vi "Stop Core.vi"(10 "final error code":i32, 11 "Example Controller Actor In":refnum<class "Example Controller Actor.lvclass">) -> (3 "Example Controller Actor Out":refnum<class "Example Controller Actor.lvclass">)   [LabVIEW 2017, in "Example GUI View Actor.lvlib" / "Example Controller Actor.lvclass"]
doc: "(<B>Filename</B>: Actor Framework.lvlib:Actor.lvclass:Stop Core.vi)\n\nDefines what the actor does before it stops. Use the <B>final error code</B> input to determine whether the actor shut down in response to an error.\n\nBy default, this method does nothing. A descendant class may override it to define behavior, such as shutting down any processes the actor initiated in its override of the Actor Core method."
uses:
  Example Controller Actor.lvclass
  Example Controller Actor.lvclass/Example Controller Actor.ctl
  Example Controller Actor/Example Controller Actor/Example Controller Actor.lvclass
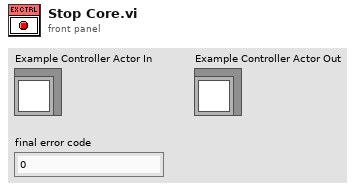
[diagram p1: front panel]
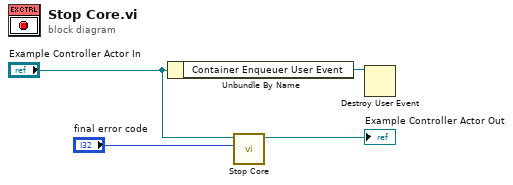
[diagram p0: block diagram]
diagram:
  n1 = Unbundle By Name("Example Controller Actor In") -> ("Container Enqueuer User Event"=w1:refnum<user-event>)
  n2 = call-parent "Stop Core.vi"("final error code"="final error code", "Controller Actor In"="Example Controller Actor In") -> ("Controller Actor Out"=→"Example Controller Actor Out":refnum<class "Example Controller Actor.lvclass">)  [unwired: 9 in]
  n3 = Destroy User Event(user event=w1) -> ()  [unwired: 1 in, 1 out]
